vi "radar_area.vi"(11 "String":string) -> (2 "area point Array":cluster{cdb[]}[](array[cluster]), 3 "areas":string[](array[string]))   [LabVIEW 2022 SP3]
panel:
  out "XY Graph":cluster{cdb[]}[](graph)
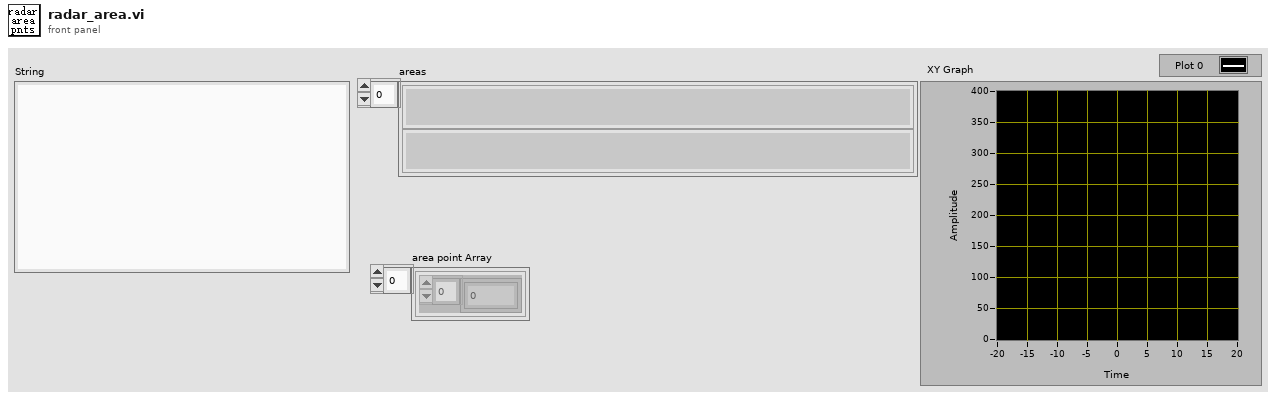
[diagram p1: front panel]
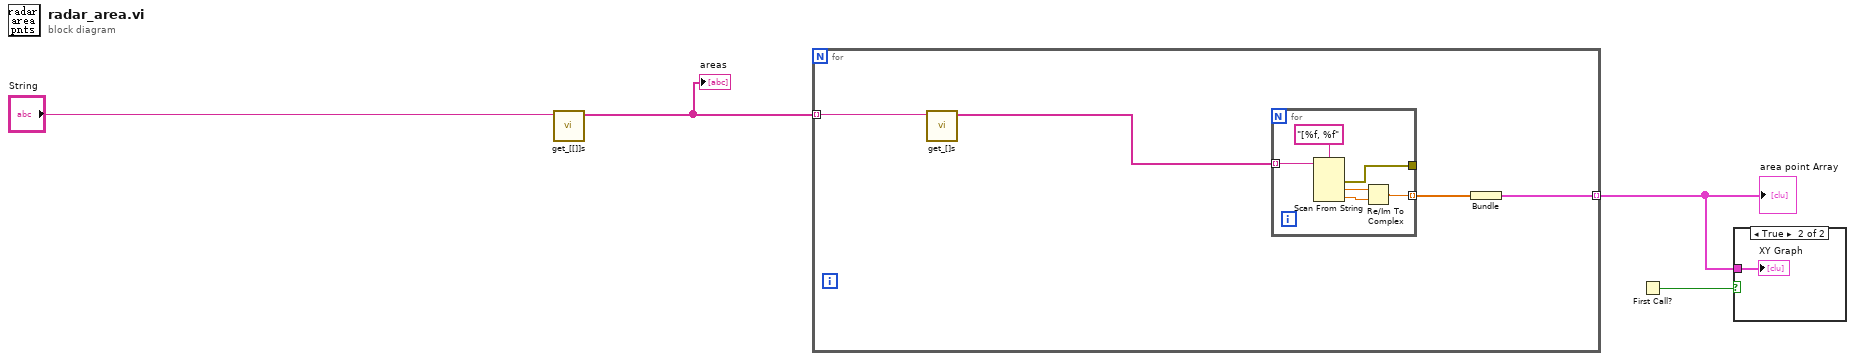
[diagram p0: block diagram]
diagram:
  n1 = call "get_[[]]s.vi"("String"="String") -> ("Array"=w4:string[])  [unwired: 10 in]
  "areas" <- w4
  n2 = for {
    tunnel: w4 -> [w8] mode=indexing
    tunnel: [w5] -> w2 mode=indexing
    n3 = call "get_[]s.vi"("String"=w8) -> ("[]Array"=w7:string[])  [unwired: 10 in]
    n4 = for {
      tunnel: w7 -> [w14] mode=indexing
      tunnel: [w12] -> w6 mode=indexing
      tunnel: [w9] -> _
      n5 = Scan From String(format string="[%f, %f", input string=w14) -> (error out=w9:errorcluster, output 1=w11:dbl, output 2=w10:dbl)  [unwired: 4 in, 2 out]
      n6 = Re/Im To Complex(1:w10, 2:w11) -> (0:w12:cdb)
    }
    n7 = Bundle(w6) -> (w5:cluster{cdb[]})  [unwired: 1 in]
  }
  "area point Array" <- w2
  n8 = First Call?() -> (First Call?: T/F=w1:bool)
  n9 = case shown="True" w1 {
    tunnel: w2 -> [_ w15]
    frame False {
    }
    frame True {
      "XY Graph" <- w15
    }
  }
